vi "Write File.vi"(8 "error in (no error)":errorcluster, 10 "Parameters":refnum<class "Parameter.lvclass">[](array[class]), 11 "Parameter INI File in":refnum<class "Parameter INI File.lvclass">) -> (0 "error out":errorcluster, 3 "Parameter INI File out":refnum<class "Parameter INI File.lvclass">)   [LabVIEW 2019, in "CD Parameter Manager API.lvlib" / "Parameter INI File.lvclass"]
uses:
  Parameter INI File.lvclass
  Parameter Class/Parameter.lvclass
  Parameter INI File.lvclass/Parameter INI File.ctl
  Double Parameter Class/Double Parameter.lvclass
  C:/Repositories/UI-Control-Initializer-API/Source/Parameter Class/Parameter.lvclass
  Parameter Class/Parameter.lvclass/Parameter.ctl
  Double Parameter Class/Double Parameter.lvclass/Double Parameter.ctl
  Boolean Parameter Class/Boolean Parameter.lvclass
  Boolean Parameter Class/Boolean Parameter.lvclass/Boolean Parameter.ctl
  I32 Parameter Class/I32 Parameter.lvclass
  I32 Parameter Class/I32 Parameter.lvclass/I32 Parameter.ctl
  String Parameter Class/String Parameter.lvclass
  String Parameter Class/String Parameter.lvclass/String Parameter.ctl
  Parameter Class/Member Accessors/Read Control label.vi
  Double Parameter Class/Member Accessors/Read Value.vi
  Boolean Parameter Class/Member Accessors/Read Value.vi
  I32 Parameter Class/Member Accessors/Read Value.vi
  String Parameter Class/Member Accessors/Read Value.vi
  <vilib>/Utility/config.llb/Write Key (Double).vi
  <vilib>/Utility/config.llb/Write Key (Boolean).vi
  <vilib>/Utility/config.llb/Write Key (I32).vi
  <vilib>/Utility/config.llb/Write Key (String).vi
  <vilib>/Utility/error.llb/Error Cluster From Error Code.vi
  <vilib>/ErrorRing/Error Ring.xnode
  <vilib>/Utility/config.llb/NI_LVConfig.lvlib
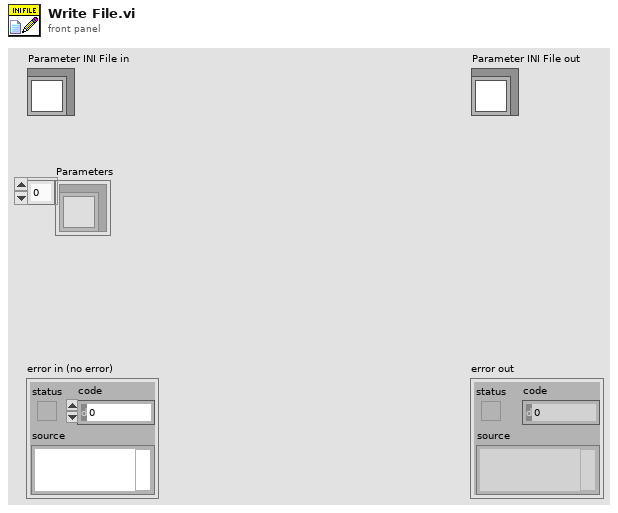
[diagram p1: front panel]
types:
  T1 = typedef "NI_LVConfig.lvlib/Config Data RefNum.ctl" = refnum<k1>
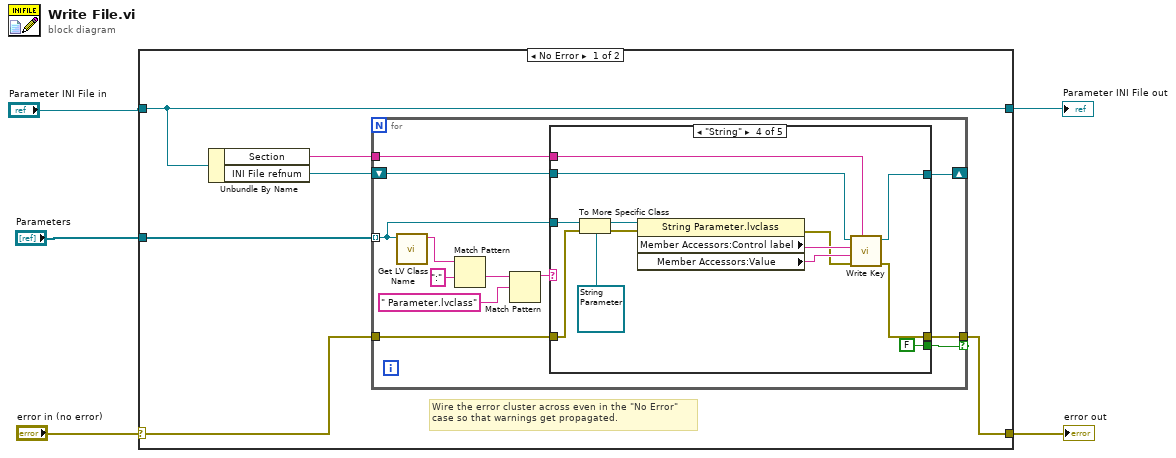
[diagram p0: block diagram]
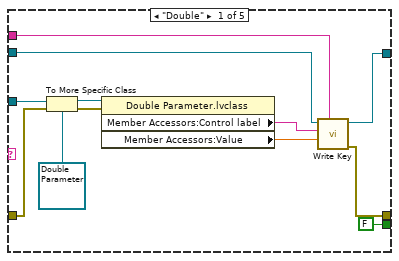
[diagram p2: hidden frame]
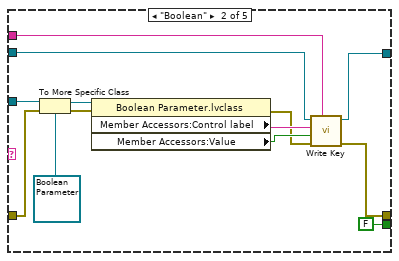
[diagram p3: hidden frame]
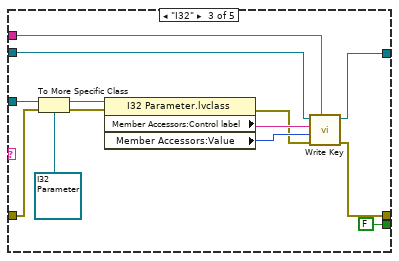
[diagram p4: hidden frame]
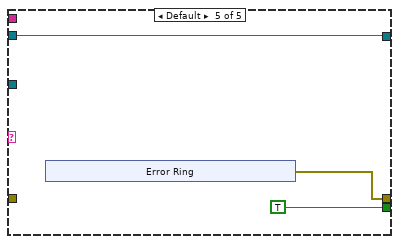
[diagram p5: hidden frame]
diagram:
  n1 = case shown="No Error" "error in (no error)" {
    selector: "error in (no error)" -> [w11 w84]
    tunnel: [w10 w84] -> w2
    tunnel: [w9 w83] -> w3
    tunnel: "Parameter INI File in" -> [w9 w83]
    tunnel: "Parameters" -> [w6 _]
    frame No Error {
      # "Wire the error cluster across even in the \"No Error\"\ncase so that warnings get propagated."
      n2 = Unbundle By Name(w9) -> ("Section"=w7:string, "INI File refnum"=w8:T1)
      n3 = for {
        tunnel: w11 -> [w18]
        tunnel: [w13] -> w10 if=w14
        tunnel: w6 -> [w16] mode=indexing
        tunnel: w7 -> [w15]
        shift-right: [w12] -> _
        shift-left: w8 -> [w17]
        n4 = call <vilib>:"Get LV Class Name.vi"("object"=w16) -> ("class name"=w20:string)  [unwired: 9 in, 1 out]
        n5 = Match Pattern(string=w20, regular expression=":") -> (after substring=w22:string)  [unwired: 1 in, 3 out]
        n6 = Match Pattern(string=w22, regular expression=" Parameter.lvclass") -> (before substring=w19:string)  [unwired: 1 in, 3 out]
        n7 = case shown="\"String\"" w19 {
          tunnel: w18 -> [w31 w43 w56 w69 _]
          tunnel: [w26 w42 w51 w65 w76] -> w13
          tunnel: [FALSE ("found?") FALSE ("found?") FALSE ("found?") FALSE ("found?") TRUE] -> w14
          tunnel: w17 -> [w27 w39 w54 w67 w75]
          tunnel: w16 -> [w34 w44 w57 w70 _]
          tunnel: w15 -> [w28 w40 w53 w66 _]
          tunnel: [w24 w36 w49 w63 w75] -> w12
          frame "Double" {
            n8 = To More Specific Class(target class=refnum<class "Double Parameter.lvclass"> refnum ("CD Parameter Manager API.lvlib:Double Parameter.lvclass"), reference=w34, error in=w31) -> (specific class reference=w33:refnum<class "Double Parameter.lvclass">, error out=w35:errorcluster)
            n9 = property class="Double Parameter.lvclass"(reference=w33, error in=w35) -> ("Member Accessors:Control label"=w29:string, "Member Accessors:Value"=w30:dbl)  [unwired: 2 out]
            n10 = call-poly <vilib>:"Write Key.vi"("section"=w28, "value"=w30, "key"=w29, "refnum"=w27) -> ("error out"=w26:errorcluster, "refnum out"=w24:T1)  [unwired: 5 in, 1 out]
          }
          frame "Boolean" {
            n11 = To More Specific Class(target class=refnum<class "Boolean Parameter.lvclass"> refnum ("CD Parameter Manager API.lvlib:Boolean Parameter.lvclass"), reference=w44, error in=w43) -> (specific class reference=w46:refnum<class "Boolean Parameter.lvclass">, error out=w47:errorcluster)
            n12 = property class="Boolean Parameter.lvclass"(reference=w46, error in=w47) -> (error out=w41:errorcluster, "Member Accessors:Control label"=w48:string, "Member Accessors:Value"=w45:bool)  [unwired: 1 out]
            n13 = call-poly <vilib>:"Write Key.vi"("section"=w40, "error in (no error)"=w41, "value"=w45, "key"=w48, "refnum"=w39) -> ("error out"=w42:errorcluster, "refnum out"=w36:T1)  [unwired: 4 in, 1 out]
          }
          frame "I32" {
            n14 = To More Specific Class(target class=refnum<class "I32 Parameter.lvclass"> refnum ("CD Parameter Manager API.lvlib:I32 Parameter.lvclass"), reference=w57, error in=w56) -> (specific class reference=w59:refnum<class "I32 Parameter.lvclass">, error out=w60:errorcluster)
            n15 = property class="I32 Parameter.lvclass"(reference=w59, error in=w60) -> (error out=w55:errorcluster, "Member Accessors:Control label"=w61:string, "Member Accessors:Value"=w58:i32)  [unwired: 1 out]
            n16 = call-poly <vilib>:"Write Key.vi"("section"=w53, "error in (no error)"=w55, "value"=w58, "key"=w61, "refnum"=w54) -> ("error out"=w51:errorcluster, "refnum out"=w49:T1)  [unwired: 4 in, 1 out]
          }
          frame "String" {
            n17 = To More Specific Class(target class=refnum<class "String Parameter.lvclass"> refnum ("CD Parameter Manager API.lvlib:String Parameter.lvclass"), reference=w70, error in=w69) -> (specific class reference=w72:refnum<class "String Parameter.lvclass">, error out=w73:errorcluster)
            n18 = property class="String Parameter.lvclass"(reference=w72, error in=w73) -> (error out=w68:errorcluster, "Member Accessors:Control label"=w74:string, "Member Accessors:Value"=w71:string)  [unwired: 1 out]
            n19 = call-poly <vilib>:"Write Key.vi"("section"=w66, "error in (no error)"=w68, "value"=w71, "key"=w74, "refnum"=w67) -> ("error out"=w65:errorcluster, "refnum out"=w63:T1)  [unwired: 4 in, 1 out]
          }
          frame Default {
            n20 = xnode "Error Ring"() -> ("error out"=w76:errorcluster)
          }
        }
      }
    }
    frame Error {
    }
  }
  "error out" <- w2
  "Parameter INI File out" <- w3
